vi "Read Electrical Variables ASCO PQM.vi"(8 "Error in":errorcluster, 11 "Modbus master in":refnum<class "Modbus Master.lvclass">) -> (0 "Error out":errorcluster, 2 "Electrical Variables":sgl[](array[numeric]), 3 "Modbus master out":refnum<class "Modbus Master.lvclass">)   [LabVIEW 2019]
uses:
  <vilib>/Modbus/master/Modbus Master.lvclass
panel:
  out "AC Average RMS Current":sgl
  out "AC L3 RMS Current":sgl format="%#.1f"
  out "AC L2 RMS Current":sgl format="%#.1f"
  out "AC L1 RMS Current":sgl format="%#.1f"
  out "Power Factor":sgl
  out "Apparent Power":sgl
  out "AC L3 Line-Neutral Voltage":sgl format="%#.1f"
  out "AC L2 Line-Neutral Voltage":sgl format="%#.1f"
  out "AC L1 Line-Neutral Voltage":sgl format="%#.1f"
  out "AC L3-L1 Line-Line Voltage":sgl format="%#.1f"
  out "AC L2-L3 Line-Line Voltage":sgl format="%#.1f"
  out "AC L1-L2 Line-Line Voltage":sgl format="%#.1f"
  out "Frequency":sgl
  out "Reactive Power":sgl
  out "Real Power":sgl
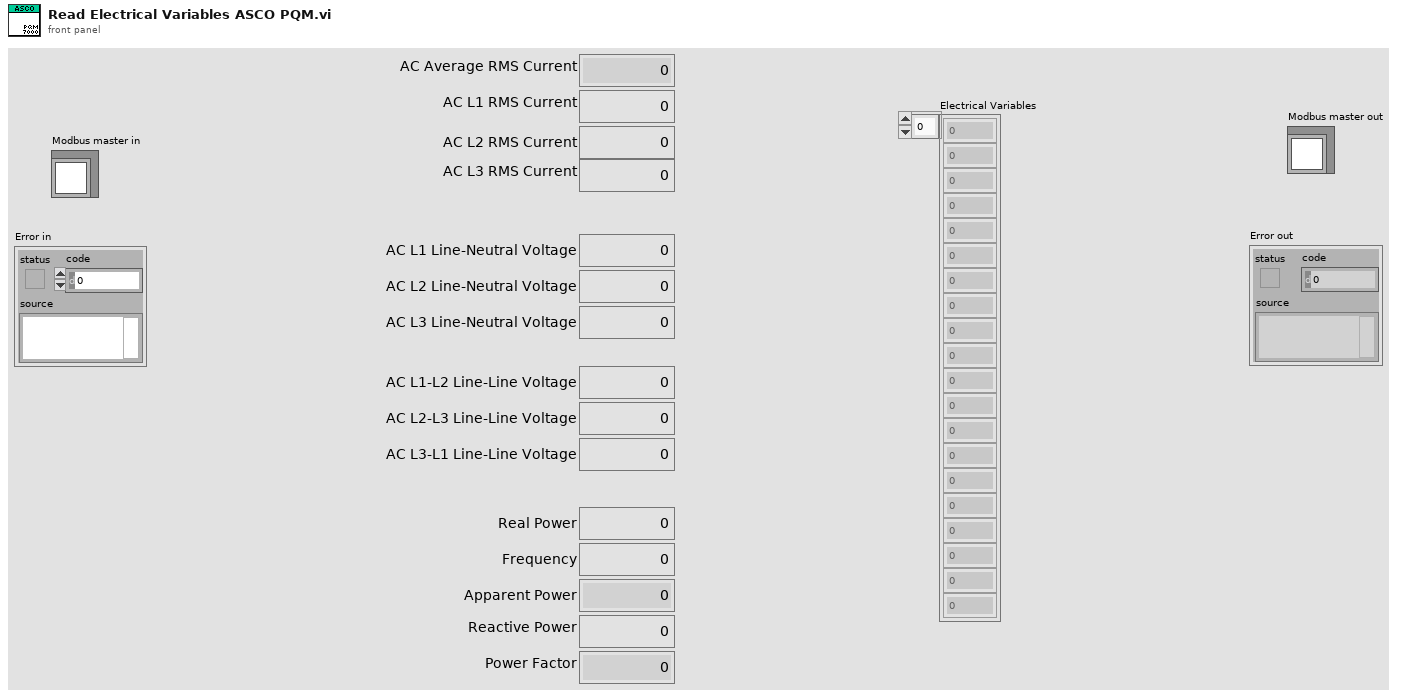
[diagram p1: front panel]
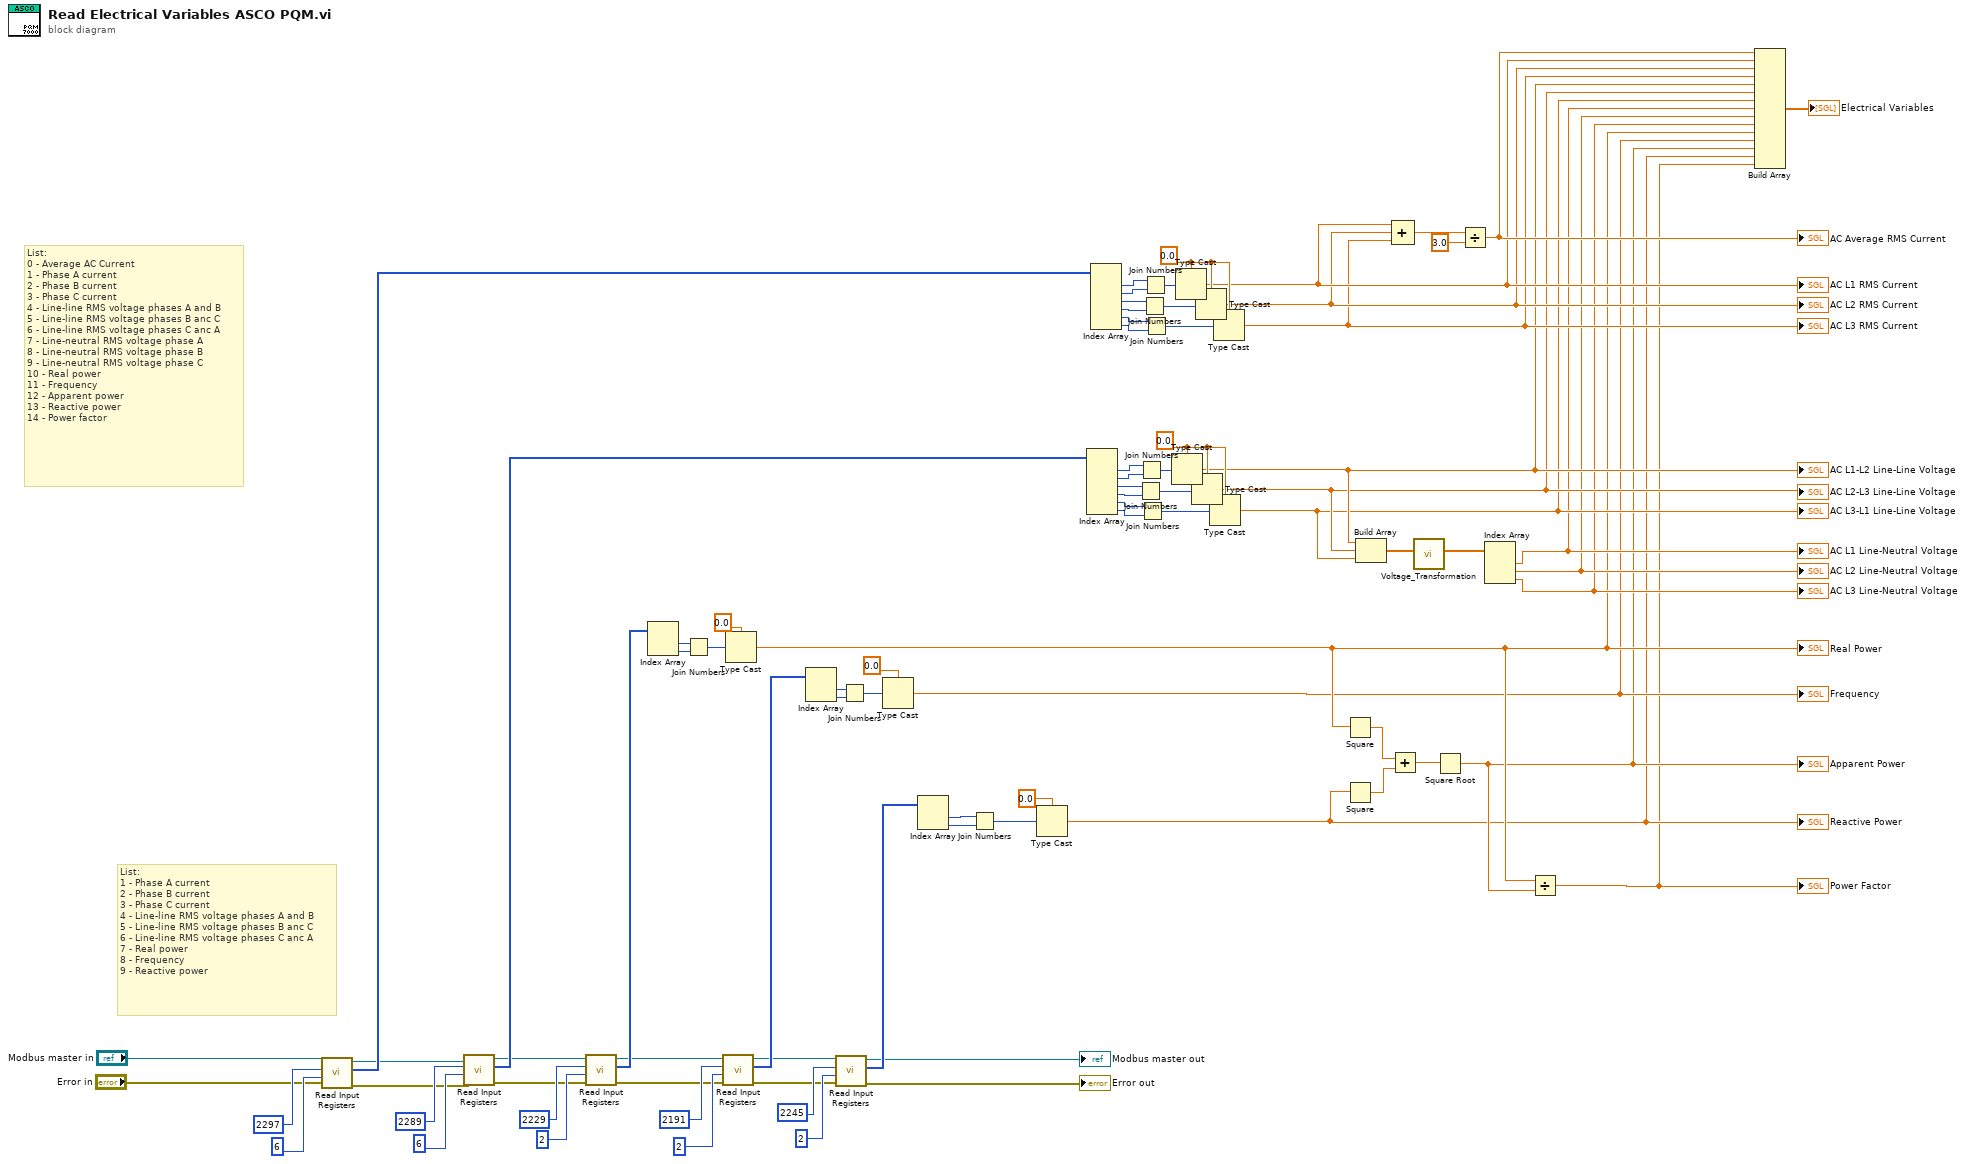
[diagram p0: block diagram]
diagram:
  w22 = sgl 0.0
  w73 = sgl 0.0
  # "List:\n1 - Phase A current\n2 - Phase B current\n3 - Phase C current\n4 - Line-line RMS voltage phases A and B\n5 - Line-line RMS voltage phases B anc C\n6 - Line-line RMS voltage phases C anc A\n7 - Real power\n8 - Frequency\n9 - Reactive power"
  # "List:\n0 - Average AC Current\n1 - Phase A current\n2 - Phase B current\n3 - Phase C current\n4 - Line-line RMS voltage phases A and B\n5 - Line-line RMS voltage phases B anc C\n6 - Line-line RMS voltage phases C anc A\n7 - Line-neutral RMS voltage phase A\n8 - Line-neutral RMS voltage phase B\n9 - Line-neutral RMS voltage phase C\n10 - Real power\n11 - Frequency\n12 - Apparent power\n13 - Reactive power\n14 - Power factor"
  n1 = call-dynamic "Read Input Registers.vi"("error in (no error)"="Error in", "number of input registers"=u16 6 ("number of holding registers"), "starting address"=u16 2297, "Modbus master in"="Modbus master in") -> ("error out"=w19:errorcluster, "register values"=w21:u16[], "Modbus master out"=w20:refnum<class "Modbus Master.lvclass">)  [unwired: 5 in]
  n2 = call-dynamic "Read Input Registers.vi"("error in (no error)"=w19, "number of input registers"=u16 6 ("number of holding registers"), "starting address"=u16 2289, "Modbus master in"=w20) -> ("error out"=w61:errorcluster, "register values"=w71:u16[], "Modbus master out"=w62:refnum<class "Modbus Master.lvclass">)  [unwired: 5 in]
  n3 = call-dynamic "Read Input Registers.vi"("error in (no error)"=w61, "number of input registers"=u16 2 ("number of holding registers"), "starting address"=u16 2229, "Modbus master in"=w62) -> ("error out"=w43:errorcluster, "register values"=w67:u16[], "Modbus master out"=w45:refnum<class "Modbus Master.lvclass">)  [unwired: 5 in]
  n4 = Index Array(array=w67) -> (element #1=w66:u16, element #2=w65:u16)  [unwired: 2 in]
  n5 = Join Numbers(hi=w66, lo=w65) -> ((hi.lo)=w64:u32)
  n6 = call-dynamic "Read Input Registers.vi"("error in (no error)"=w43, "number of input registers"=u16 2 ("number of holding registers"), "starting address"=u16 2191, "Modbus master in"=w45) -> ("error out"=w41:errorcluster, "register values"=w48:u16[], "Modbus master out"=w42:refnum<class "Modbus Master.lvclass">)  [unwired: 5 in]
  n7 = Type Cast(type=sgl 0.0, x=w64) -> (*(type *) &x=w6:sgl)
  "Real Power" <- w6
  n8 = Index Array(array=w48) -> (element #1=w52:u16, element #2=w51:u16)  [unwired: 2 in]
  n9 = call-dynamic "Read Input Registers.vi"("error in (no error)"=w41, "number of input registers"=u16 2 ("number of holding registers"), "starting address"=u16 2245, "Modbus master in"=w42) -> ("error out"=→"Error out":errorcluster, "register values"=w58:u16[], "Modbus master out"=→"Modbus master out":refnum<class "Modbus Master.lvclass">)  [unwired: 5 in]
  n10 = Join Numbers(hi=w52, lo=w51) -> ((hi.lo)=w50:u32)
  n11 = Type Cast(type=sgl 0.0, x=w50) -> (*(type *) &x=w5:sgl)
  "Frequency" <- w5
  n12 = Index Array(array=w58) -> (element #1=w57:u16, element #2=w56:u16)  [unwired: 2 in]
  n13 = Join Numbers(hi=w57, lo=w56) -> ((hi.lo)=w54:u32)
  n14 = Type Cast(type=sgl 0.0, x=w54) -> (*(type *) &x=w3:sgl)
  "Reactive Power" <- w3
  n15 = Index Array(array=w71) -> (element #1=w82:u16, element #2=w81:u16, element #3=w80:u16, element #4=w79:u16, element #5=w78:u16, element #6=w77:u16)  [unwired: 6 in]
  n16 = Index Array(array=w21) -> (element #1=w31:u16, element #2=w30:u16, element #3=w29:u16, element #4=w28:u16, element #5=w27:u16, element #6=w26:u16)  [unwired: 6 in]
  n17 = Join Numbers(hi=w80, lo=w79) -> ((hi.lo)=w75:u32)
  n18 = Join Numbers(hi=w82, lo=w81) -> ((hi.lo)=w76:u32)
  n19 = Join Numbers(hi=w78, lo=w77) -> ((hi.lo)=w74:u32)
  n20 = Join Numbers(hi=w29, lo=w28) -> ((hi.lo)=w24:u32)
  n21 = Join Numbers(hi=w31, lo=w30) -> ((hi.lo)=w25:u32)
  n22 = Join Numbers(hi=w27, lo=w26) -> ((hi.lo)=w23:u32)
  n23 = Type Cast(type=w73, x=w76) -> (*(type *) &x=w12:sgl)
  "AC L1-L2 Line-Line Voltage" <- w12
  n24 = Type Cast(type=w22, x=w25) -> (*(type *) &x=w15:sgl)
  "AC L1 RMS Current" <- w15
  n25 = Type Cast(type=w73, x=w75) -> (*(type *) &x=w11:sgl)
  "AC L2-L3 Line-Line Voltage" <- w11
  n26 = Type Cast(type=w22, x=w24) -> (*(type *) &x=w14:sgl)
  "AC L2 RMS Current" <- w14
  n27 = Type Cast(type=w73, x=w74) -> (*(type *) &x=w10:sgl)
  "AC L3-L1 Line-Line Voltage" <- w10
  n28 = Type Cast(type=w22, x=w23) -> (*(type *) &x=w13:sgl)
  "AC L3 RMS Current" <- w13
  n29 = Square(x=w6) -> (x^2=w40:sgl)
  n30 = Square(x=w3) -> (x^2=w39:sgl)
  n31 = Build Array(w12, w11, w10) -> (w47:sgl[])
  n32 = Add(x=w40, y=w39) -> (x+y=w38:sgl)
  n33 = Compound Arithmetic op=ADD(w15, w14, w13) -> (w18:sgl)
  n34 = call "Voltage_Transformation.vi"("VLL"=w47) -> ("VLN"=w46:sgl[])  [unwired: 10 in]
  n35 = Square Root(x=w38) -> (sqrt(x)=w4:sgl)
  "Apparent Power" <- w4
  n36 = Divide(x=w18, y=sgl 3.0) -> (x/y=w16:sgl)
  "AC Average RMS Current" <- w16
  n37 = Index Array(array=w46) -> (element #1=w9:sgl, element #2=w8:sgl, element #3=w7:sgl)  [unwired: 3 in]
  "AC L1 Line-Neutral Voltage" <- w9
  "AC L2 Line-Neutral Voltage" <- w8
  "AC L3 Line-Neutral Voltage" <- w7
  n38 = Divide(x=w6, y=w4) -> (x/y=w2:sgl)
  "Power Factor" <- w2
  n39 = Build Array(w16, w15, w14, w13, w12, w11, w10, w9, w8, w7, w6, w5, w4, w3, w2) -> (→"Electrical Variables":sgl[])
